vi "Path to front panel.vi"(8 "error in (no error)":errorcluster, 11 "PS Control Persistence Actor in":refnum<class "PS Control Persistence Actor.lvclass">) -> (0 "error out":errorcluster, 2 "Path to front panel VI":path, 3 "PS Control Persistence Actor out":refnum<class "PS Control Persistence Actor.lvclass">)   [LabVIEW 2024, in "PS Control Persistence.lvlib" / "PS Control Persistence Actor.lvclass"]
uses:
  PS Control Persistence Actor.lvclass
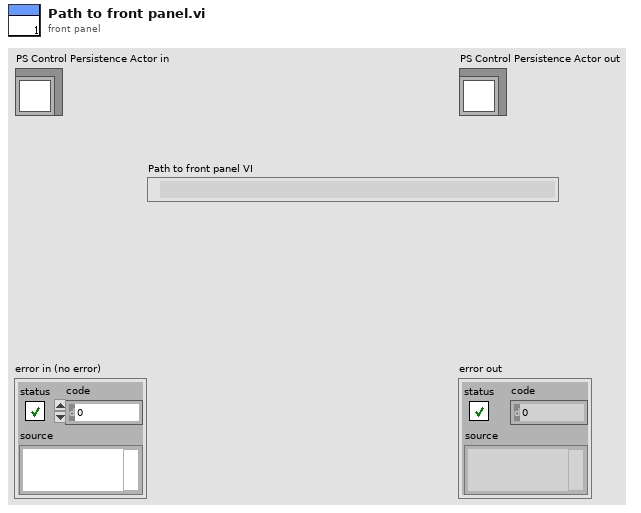
[diagram p1: front panel]
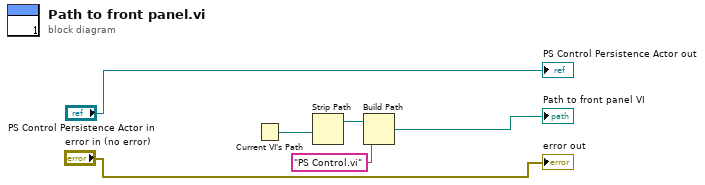
[diagram p0: block diagram]
diagram:
  n1 = Current VI's Path() -> (path=w6:path)
  n2 = Strip Path(path=w6) -> (stripped path=w5:path)  [unwired: 1 out]
  n3 = Build Path(base path=w5, name or relative path="PS Control.vi") -> (appended path=→"Path to front panel VI":path)
  "error out" <- "error in (no error)"
  "PS Control Persistence Actor out" <- "PS Control Persistence Actor in"
